vi "File Details.vi"(0 "Path":path, 5 "File/Folder Name":string, 11 "Error In":errorcluster) -> (8 "Report":string, 15 "error out":errorcluster)   [LabVIEW 2020, in "File explorer 2.0.lvlib"]
doc: "This VI is used as a subVI which is used to extract the data from the tree file hierarchy."
uses:
  File explorer 2.0.lvlib
panel:
  # "FILE DETAILS EXTRACTION VI"
  # "Extracting the details of the file like last modified, size and file type"
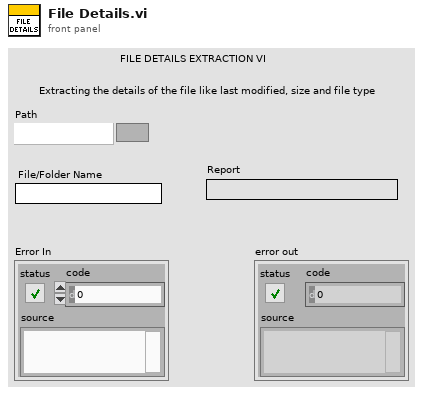
[diagram p1: front panel]
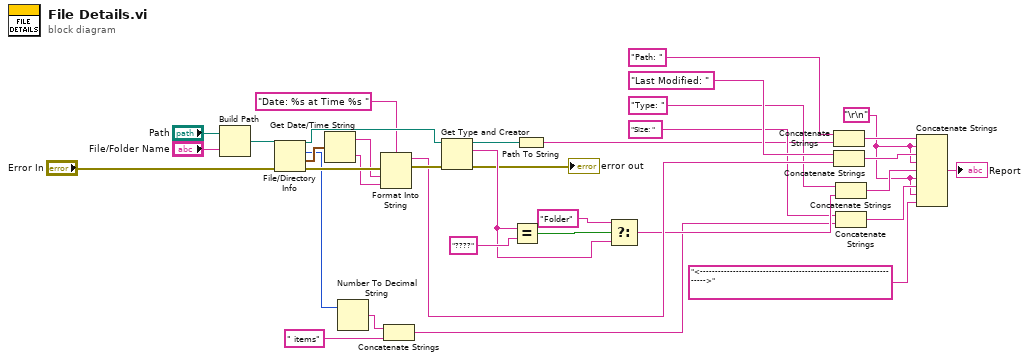
[diagram p0: block diagram]
diagram:
  w5 = "\r\n"
  n1 = Build Path(base path="Path", name or relative path="File/Folder Name") -> (appended path=w33:path)
  n2 = File/Directory Info(path=w33, error in="Error In") -> (path out=w35:path, size=w24:i64, last mod=w27:timestamp, error out=w28:errorcluster)  [unwired: 3 out]
  n3 = Get Date/Time String(seconds (now)=w27) -> (date string=w26:string, time string=w25:string)  [unwired: 2 in]
  n4 = Number To Decimal String(number=w24) -> (decimal integer string=w23:string)  [unwired: 1 in]
  n5 = Format Into String(format string="Date: %s at Time %s ", error in=w28, w26, w25) -> (resulting string=w16:string, error out=w34:errorcluster)  [unwired: 1 in]
  n6 = Concatenate Strings(w23, " items" ("string")) -> (w12:string)
  n7 = Get Type and Creator(4:w34, 7:w35) -> (0:→"error out":errorcluster, 2:w19:string, 3:w22:path)  [unwired: 1 out]
  n8 = Equal?(x=w19, y="????") -> (x = y?=w20:bool)
  n9 = Path To String(path=w22) -> (string=w10:string)
  n10 = Select(t="Folder", s=w20, f=w19) -> (s? t:f=w14:string)
  n11 = Concatenate Strings("Path: " ("string"), w10) -> (w9:string)
  n12 = Concatenate Strings("Last Modified: " ("string"), w16) -> (w8:string)
  n13 = Concatenate Strings("Type: " ("string"), w14) -> (w7:string)
  n14 = Concatenate Strings("Size: " ("string"), w12) -> (w6:string)
  n15 = Concatenate Strings(w9, w5, w8, w5, w7, w5, w6, w5, "<-------------------------------------------------------------------->" ("string")) -> (→"Report":string)
